vi "To Generic.vi"(8 "error in (no error)":errorcluster, 11 "Request Data in":refnum<class "Multi Data.lvclass">) -> (0 "error out":errorcluster, 2 "Generic Data":refnum<class "Generic Data.lvclass">[](array[class]), 3 "Data Name":string[](array[string]))   [LabVIEW 2020, in "Publisher.lvlib" / "Multi Data.lvclass"]
doc: "Present private data as an array of named generic data elements.\n\nThis implementation uses the Data Alias Array as prefixes if and only if it has the same size as the Data Array. If the Data Alias Array is not used the regular Data Alias is used instead."
uses:
  Multi Data.lvclass
  PPL/HDH.Data.Generic.lvlibp/Generic Data/Generic Data.lvclass
  Multi Data.lvclass/Multi Data.ctl
  Timed Data/Timed Data.lvclass
  PPL/HDH.Data.Generic.lvlibp/Data.lvclass
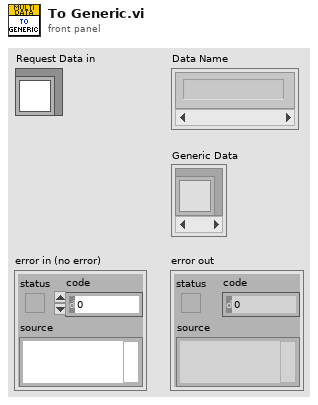
[diagram p1: front panel]
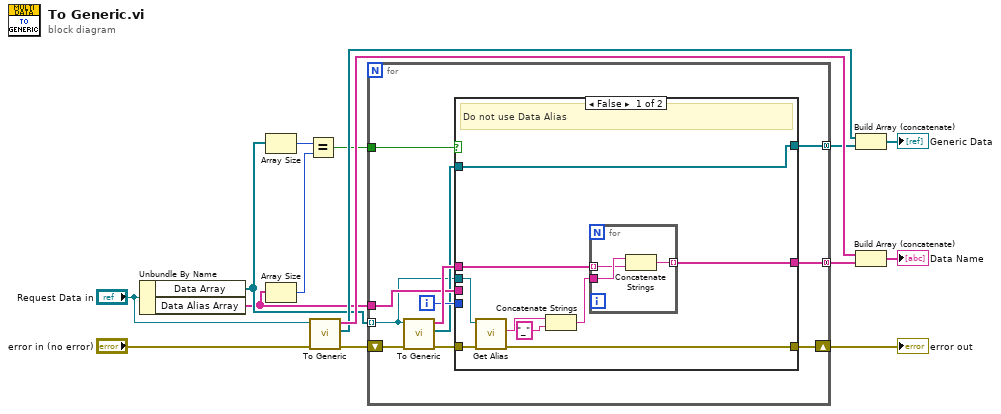
[diagram p0: block diagram]
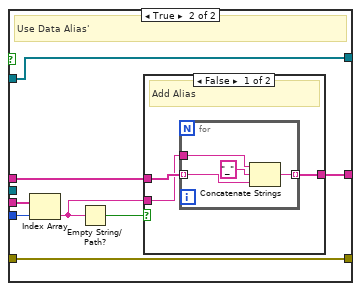
[diagram p2: hidden frame]
diagram:
  n1 = Unbundle By Name("Request Data in") -> ("Data Array"=w7:refnum<class "Data.lvclass">[], "Data Alias Array"=w5:string[])
  n2 = Array Size(array=w7) -> (size(s)=w9:i32)
  n3 = Array Size(array=w5) -> (size(s)=w8:i32)
  n4 = Equal?(x=w9, y=w8) -> (x = y?=w6:bool)
  n5 = call-parent "To Generic.vi"("error in (no error)"="error in (no error)", "Request Data in"="Request Data in") -> ("error out"=w4:errorcluster, "Generic Data"=w14:refnum<class "Generic Data.lvclass">[], "Data Name"=w15:string[])  [unwired: 7 in]
  n6 = for {
    tunnel: w7 -> [w21] mode=indexing
    tunnel: w6 -> [w26]
    tunnel: w5 -> [w24]
    shift-right: [w19] -> w3
    shift-left: w4 -> [w20]
    tunnel: [w17] -> w2 mode=concatenating
    tunnel: [w16] -> w1 mode=concatenating
    i -> [w23]
    n7 = call-dynamic "To Generic.vi"("error in (no error)"=w20, "Data in"=w21) -> ("error out"=w18:errorcluster, "Generic Data"=w22:refnum<class "Generic Data.lvclass">[], "Data Name"=w25:string[])  [unwired: 7 in]
    n8 = case shown="False" w26 {
      tunnel: w25 -> [w33 w44]
      tunnel: w24 -> [_ w45]
      tunnel: w23 -> [_ w46]
      tunnel: w22 -> [w28 w43]
      tunnel: [w28 w43] -> w17
      tunnel: [w29 w42] -> w16
      tunnel: w21 -> [w35 _]
      tunnel: [w27 w39] -> w19
      tunnel: w18 -> [w34 w39]
      frame False {
        # "Do not use Data Alias"
        n9 = call-dynamic "Get Alias.vi"("error in (no error)"=w34, "Data in"=w35) -> ("error out"=w27:errorcluster, "Alias"=w32:string)  [unwired: 7 in, 1 out]
        n10 = Concatenate Strings(w32, "_" ("string")) -> (w30:string)
        n11 = for {
          tunnel: w33 -> [w37] mode=indexing
          tunnel: w30 -> [w38]
          tunnel: [w36] -> w29 mode=indexing
          n12 = Concatenate Strings(w38, w37) -> (w36:string)
        }
      }
      frame True {
        # "Use Data Alias'"
        n13 = Index Array(array=w45, index=w46) -> (element=w41:string)
        n14 = Empty String/Path?(string/path=w41) -> (empty?=w40:bool)
        n15 = case shown="False" w40 {
          tunnel: w44 -> [w49 w54]
          tunnel: [w48 w54] -> w42
          tunnel: w41 -> [w47 _]
          frame False {
            # "Add Alias"
            n16 = for {
              tunnel: w47 -> [w53]
              tunnel: w49 -> [w51] mode=indexing
              tunnel: [w50] -> w48 mode=indexing
              n17 = Concatenate Strings(w53, "_" ("string"), w51) -> (w50:string)
            }
          }
          frame True {
            # "Empty Alias - Add nothing"
          }
        }
      }
    }
  }
  "error out" <- w3
  n18 = Build Array (concatenate)(w14, w2) -> (→"Generic Data":refnum<class "Generic Data.lvclass">[])
  n19 = Build Array (concatenate)(w15, w1) -> (→"Data Name":string[])
